vi "Serve Buffer to Connection.vi"(7 "framework period":u32 format="%d us", 8 "error in (no error)":errorcluster, 9 "Status":refnum<class "Status Pointer.lvclass">, 10 "Buffer":refnum<class "Buffer.lvclass">, 11 "connection ID in":refnum<k5>) -> (0 "error out":errorcluster, 3 "connection ID out":refnum<k5>)   [LabVIEW 2017, in "DSF Core.lvlib" / "Data Server Thread.lvclass"]
uses:
  Data Server Thread.lvclass
  Buffer/Buffer.lvclass
  C:/Program Files (x86)/National Instruments/LabVIEW 2017/vi.lib/NI/Memory Manager/Classes/Pointer/Pointer.lvclass
  Status/Status Pointer.lvclass
  <vilib>/NI/Memory Manager/Classes/Pointer/Pointer.lvclass/Pointer.ctl
  DSF Performance Metrics.ctl
  <vilib>/NI/Memory Manager/Classes/Pointer/Get Address.vi
  <vilib>/NI/Memory Manager/Classes/Pointer/Pointer.lvclass
  DSF Core.lvlib
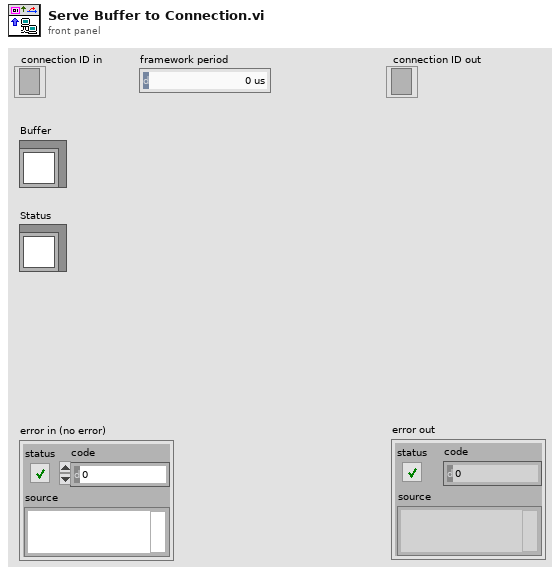
[diagram p1: front panel]
types:
  T1 = enum16{"big-endian, network order", "native, host order", "little-endian"}
  T2 = typedef "DSF Core.lvlib/DSF Performance Metrics.ctl" = cluster{"framework period":u32, "iteration":u64, "late count":u64, "duration":u64}
  T3 = typedef "DSF Core.lvlib/Status Pointer.lvclass/Status Data.ctl" = cluster{"duration":u64, "period":u64, "iteration":u64, "late count":u64}
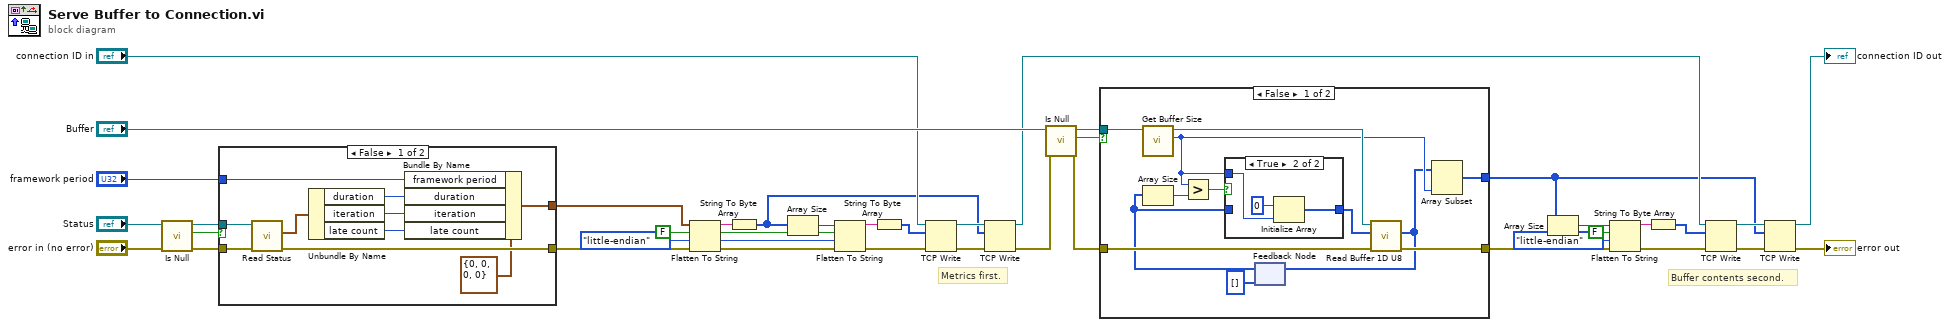
[diagram p0: block diagram]
diagram:
  w25 = T1."little-endian" ("byte order (0:big-endian, network order)")
  w26 = FALSE ("prepend array or string size? (T)")
  # "Buffer contents second."
  # "Metrics first."
  n1 = call <vilib>:"Is Null.vi"("error in (no error)"="error in (no error)", "Pointer in"="Status") -> ("error out"=w33:errorcluster, "null?"=w32:bool, "Pointer out"=w31:refnum<class "Status Pointer.lvclass">)  [unwired: 7 in]
  n2 = case shown="False" w32 {
    tunnel: w33 -> [w47 w49]
    tunnel: w31 -> [w48 _]
    tunnel: [w43 w49] -> w21
    tunnel: "framework period" -> [w40 _]
    tunnel: [w42 _] -> w19
    frame False {
      n3 = call "Read Status.vi"("error in (no error)"=w47, "status pointer in"=w48) -> ("error out"=w43:errorcluster, "status"=w46:T3)  [unwired: 7 in, 1 out]
      n4 = Unbundle By Name(w46) -> ("duration"=w39:u64, "iteration"=w45:u64, "late count"=w44:u64)
      n5 = Bundle By Name(cluster=T2 {"framework period"=0, "iteration"=0, "late count"=0, "duration"=0} ("metrics"), "framework period"=w40, "duration"=w39, "iteration"=w45, "late count"=w44) -> (w42:T2)
    }
    frame True {
    }
  }
  n6 = Flatten To String(anything=w19, prepend array or string size? (T)=w26, byte order (0:big-endian, network order)=w25, error in (no error)=w21) -> (data string=w17:string, error out=w27:errorcluster)  [unwired: 1 out]
  n7 = String To Byte Array(string=w17) -> (unsigned byte array=w3:u8[])
  n8 = Array Size(array=w3) -> (size(s)=w24:i32)
  n9 = Flatten To String(anything=w24, prepend array or string size? (T)=w26, byte order (0:big-endian, network order)=w25, error in (no error)=w27) -> (data string=w2:string, error out=w23:errorcluster)  [unwired: 1 out]
  n10 = String To Byte Array(string=w2) -> (unsigned byte array=w1:u8[])
  n11 = TCP Write(connection ID="connection ID in", data in=w1, error in (no error)=w23) -> (connection ID out=w28:refnum<k5>, error out=w29:errorcluster)  [unwired: 1 in, 1 out]
  n12 = TCP Write(connection ID=w28, data in=w3, error in (no error)=w29) -> (connection ID out=w7:refnum<k5>, error out=w20:errorcluster)  [unwired: 1 in, 1 out]
  n13 = call <vilib>:"Is Null.vi"("error in (no error)"=w20, "Pointer in"="Buffer") -> ("error out"=w37:errorcluster, "null?"=w36:bool, "Pointer out"=w38:refnum<class "Buffer.lvclass">)  [unwired: 7 in]
  n14 = case shown="False" w36 {
    tunnel: [w52 w66] -> w10
    tunnel: w38 -> [w56 _]
    tunnel: w37 -> [w55 w66]
    tunnel: [w50 _] -> w6
    frame False {
      n15 = call "Get Buffer Size.vi"("Buffer in"=w56) -> ("buffer size"=w53:u64, "Buffer out"=w57:refnum<class "Buffer.lvclass">)  [unwired: 9 in]
      n16 = feedback #1(u8[] []) -> (w54:u8[])
      n17 = Array Size(array=w54) -> (size(s)=w60:i32)
      n18 = Greater?(x=w53, y=w60) -> (0:w59:bool)
      n19 = case shown="True" w59 {
        tunnel: [w62 w64] -> w58
        tunnel: w54 -> [w62 _]
        tunnel: w53 -> [_ w63]
        frame False {
        }
        frame True {
          n20 = Initialize Array(u8 0, w63) -> (w64:u8[])
        }
      }
      n21 = call "Read Buffer 1D U8.vi"("error in (no error)"=w55, "dst array in"=w58, "Buffer in"=w57) -> ("error out"=w52:errorcluster, "dst array out"=w51:u8[])  [unwired: 5 in, 2 out]
      n22 = feedback-in #1(w51) -> ()
      n23 = Array Subset(array=w51, length=w53) -> (w50:u8[])  [unwired: 1 in]
    }
    frame True {
    }
  }
  n24 = Array Size(array=w6) -> (size(s)=w13:i32)
  n25 = Flatten To String(anything=w13, prepend array or string size? (T)=FALSE, byte order (0:big-endian, network order)=T1."little-endian", error in (no error)=w10) -> (data string=w5:string, error out=w12:errorcluster)  [unwired: 1 out]
  n26 = String To Byte Array(string=w5) -> (unsigned byte array=w4:u8[])
  n27 = TCP Write(connection ID=w7, data in=w4, error in (no error)=w12) -> (connection ID out=w15:refnum<k5>, error out=w16:errorcluster)  [unwired: 1 in, 1 out]
  n28 = TCP Write(connection ID=w15, data in=w6, error in (no error)=w16) -> (connection ID out=→"connection ID out":refnum<k5>, error out=→"error out":errorcluster)  [unwired: 1 in, 1 out]
